vi "FPGA Main High Throughput.vi"() -> ()   [LabVIEW 2015]
doc: "The myRIO v1.1 FPGA Shipping Personality. This personality contains support for:\n- 1 Button\n- 4 LED\n- 6 Analog Input channels with 1 Sample\n- 1 Analog Input channel with N Samples\n- 4 Analog Output channels with 1 Sample\n- 1 Analog Output channel with N Samples\n- 24 Digital I/O channels with 1 Sample\n- 1 Digital Input channel with N Samples\n- 1 Digital Output channel with N Samples"
uses:
  Sub VIs/Utilities/Start Boolean.ctl
  <vilib>/Platform/TimedLoop/XDataNode/timing_clust.ctl
  <vilib>/Platform/TimedLoop/XDataNode/nitl_modes.ctl
  <vilib>/Platform/TimedLoop/XDataNode/wakeup.ctl
  <vilib>/rvi/eio/common/nirviEmuReportErrorAndStop.vi
  <vilib>/rvi/interface/RandomDataEmulation/niFpgaRandomDataHandleErrors.vi
  <vilib>/rvi/Emulation/niFpgaProcessEmulError.vi
  <vilib>/rvi/FIFO/Fifo_Resource/nirvififoEmulationSetSize.vi
  <vilib>/rvi/DataTransferAndStorage/Container/Common/niFpgaContainerGetUniqueNameForEmu.vi
  <vilib>/rvi/FIFO/Fifo_Resource/nirviFifoEmulationQueueMgr.vi
  <instcachedir>/0/nirviFifoEmulationQueueMgr_E5CAEC123FF24DC58D834DCA3CDAA9B5.lvgen/nirviFifoEmulationQueueMgr_E5CAEC123FF24DC58D834DCA3CDAA9B5_003.vi
  <vilib>/rvi/Emulation/niFpgaEmulationIsFPGAContextNoSignature.vi
  <vilib>/rvi/errors/nirviReportUnexpectedCaseInternalError.vi
  <vilib>/rvi/errors/nirviReportUnexpectedCaseInternalError (U32).vi
  <vilib>/rvi/occurrence/nirviWaitOnOccurrenceBase.vi
  <vilib>/rvi/FIFO/Fifo_Resource/nirvififoEmulationReleaseLock.vi
  <vilib>/rvi/FIFO/Fifo_Resource/nirvififoEmulationObtainLock.vi
  <vilib>/rvi/FIFO/Fifo_Resource/nirvififoEmulationCreateLock.vi
  <vilib>/Utility/error.llb/Clear Errors.vi
  <vilib>/rvi/errors/niFpgaSetErrorForExecOnDevCompSimple.vi
  <vilib>/rvi/Emulation/niFpgaSctlEmulationGetInTimedLoop.vi
  <vilib>/rvi/FIFO/Fifo_Resource/nirvififoEmulationDetermineInputValidOut.vi
  <vilib>/rvi/DataTransferAndStorage/Container/Common/niFpgaContainerExecOnDevCompGetState.vi
  <vilib>/rvi/DataTransferAndStorage/Container/Common/niFpgaContainerSetEmuInfo.vi
  <vilib>/rvi/Emulation/niFpgaCriticalErrorInLSC.vi
  <vilib>/rvi/Emulation/niFpgaGetClockAttributes.vi
  <vilib>/rvi/Emulation/niFpgaEmulationReportErrorSimple.vi
  <vilib>/rvi/eio/common/nirviEmuTemplateMethod_errors.vi
  <vilib>/Platform/TimedLoop/XDataNode/XDataNode.xnode
  <vilib>/rvi/DataTransferAndStorage/Container/XNode/niFpgaContainer.xnode
  <vilib>/rvi/FIFO/Fifo_Resource/niFpgaFifoEmulationRefIn.vi
  <vilib>/rvi/LocalResourceManager/LocalResourceManager.xnode
  <vilib>/eio/EIONode/EIONode.xnode
  <vilib>/rvi/interface/RandomDataEmulation/nirviRandomDataFpgaReadWriteTemplate.vi
  <vilib>/rvi/FIFO/Fifo_Resource/nirvififoEmulationWrite.vi
  <vilib>/rvi/FIFO/Fifo_Resource/nirvififoEmulationRead.vi
  <vilib>/Platform/TimedLoop/XDataNode/XDNodeRunTimeDep.lvlib
panel:
  out "AI.B_0.VAL":u16
  out "AI.B_1.VAL":u16
  out "AI.B_2.VAL":u16
  out "AI.B_3.VAL":u16
  in  "AO.B_1.VAL":u16
  in  "AO.B_0.VAL":u16
  out "DIO.B_15:8.IN":u8 format="%08b"
  in  "DIO.B_15:8.DIR":u8 format="%08b"
  in  "DIO.B_15:8.OUT":u8 format="%08b"
  out "DIO.B_7:0.IN":u8 format="%08b"
  in  "DIO.B_7:0.DIR":u8 format="%08b"
  in  "DIO.B_7:0.OUT":u8 format="%08b"
  in  "SYS.SELECTB":u8 format="%08b"
  in  "DO.A_1.IRQ.SELECT":bool
  in  "AO.AudioOut.IRQ.SELECT":bool
  in  "AO.A_0.IRQ.SELECT":bool
  in  "AO.A_0.VAL":u16
  out "AO.A_0.IDL":bool
  out "AO.SYS.STAT":bool
  in  "AO.SYS.GO":T1
  in  "AO.A_1.VAL":u16
  out "AI.AudioIn.IDL":bool
  out "AI.A_0.VAL":u16
  out "AI.AudioIn_R.VAL":u16
  out "AI.AudioIn_L.VAL":u16
  out "AI.A_3.VAL":u16
  out "AI.A_2.VAL":u16
  out "AI.A_1.VAL":u16
  in  "DO.A_1.ClockDivisor":u16 caption="AO LoopRate(Ticks)"
  in  "DI.A_0.ClockDivisor":u16 caption="AO LoopRate(Ticks)"
  out "DO.A_1.IDL":bool
  in  "DI.A_0.ENA":bool
  out "DI.A_0.IDL":bool
  out "DIO.A_15:8.IN":u8 format="%08b"
  in  "DIO.A_15:8.DIR":u8 format="%08b"
  in  "DIO.A_15:8.OUT":u8 format="%08b"
  out "DIO.A_7:0.IN":u8 format="%08b"
  in  "DIO.A_7:0.DIR":u8 format="%08b"
  in  "DIO.A_7:0.OUT":u8 format="%08b"
  in  "AI.AudioIn.SampleRate":u32=40000 caption="Count(Ticks)"
  out "AO.AudioOut.IDL":bool
  in  "AO.AudioOut.SampleRate":u32=40000 caption="AO LoopRate(Ticks)"
  in  "AO.AudioOut_L.VAL":u16
  in  "AO.AudioOut_R.VAL":u16
  out "AI.A_0.IDL":bool
  in  "AI.A_0.SampleRate":u32=40000 caption="Count(Ticks)"
  out "SYS.AI.RDY":bool
  in  "AO.A_0.SampleRate":u32=40000 caption="AO LoopRate(Ticks)"
  out "SYS.RDY":bool
  out "SYS.AUDIN.RDY":bool
  out "SYS.BLOCK.A/AI0.RDY":bool
  in  "SYS.SELECTA":u8 format="%08b"
  out "AI.C_0.VAL":u16
  out "AI.C_1.VAL":u16
  in  "AO.C_0.VAL":u16
  in  "AO.C_1.VAL":u16
  in  "DIO.C_7:0.OUT":u8 format="%08b"
  in  "DIO.C_7:0.DIR":u8 format="%08b"
  out "DIO.C_7:0.IN":u8 format="%08b"
  in  "SYS.SELECTC":u8 format="%08b"
  out "DI.BTN":u8 format="%08b"
  in  "DO.LED3:0":u8 format="%04b"
  out "ACC.X.VAL":u16
  out "ACC.Y.VAL":u16
  out "SYS.ACC.RDY":bool
  out "ACC.Z.VAL":u16
  # "System"
  # "Audio Connector"
  # "Onboard Devices"
  # "Connector A"
  # "Connector B"
  # "Connector C"
  # "Accelerometer"
  # "Audio Input"
  # "Analog Input"
  # "Analog Output"
  # "Digital I/O"
  # "Analog Input"
  # "Analog Output"
  # "Digital I/O"
  # "Analog Input"
  # "Analog Output"
  # "Digital I/O"
  # "Audio Block Input"
  # "Analog Block Output"
  # "Buttons & LEDs"
  # "IO Configuration"
  # "Analog Block Input"
  # "IO Configuration"
  # "Digital Block Input"
  # "Audio Output"
  # "Digital Block Output"
  # "Audio Block Output"
  # "IO Configuration"
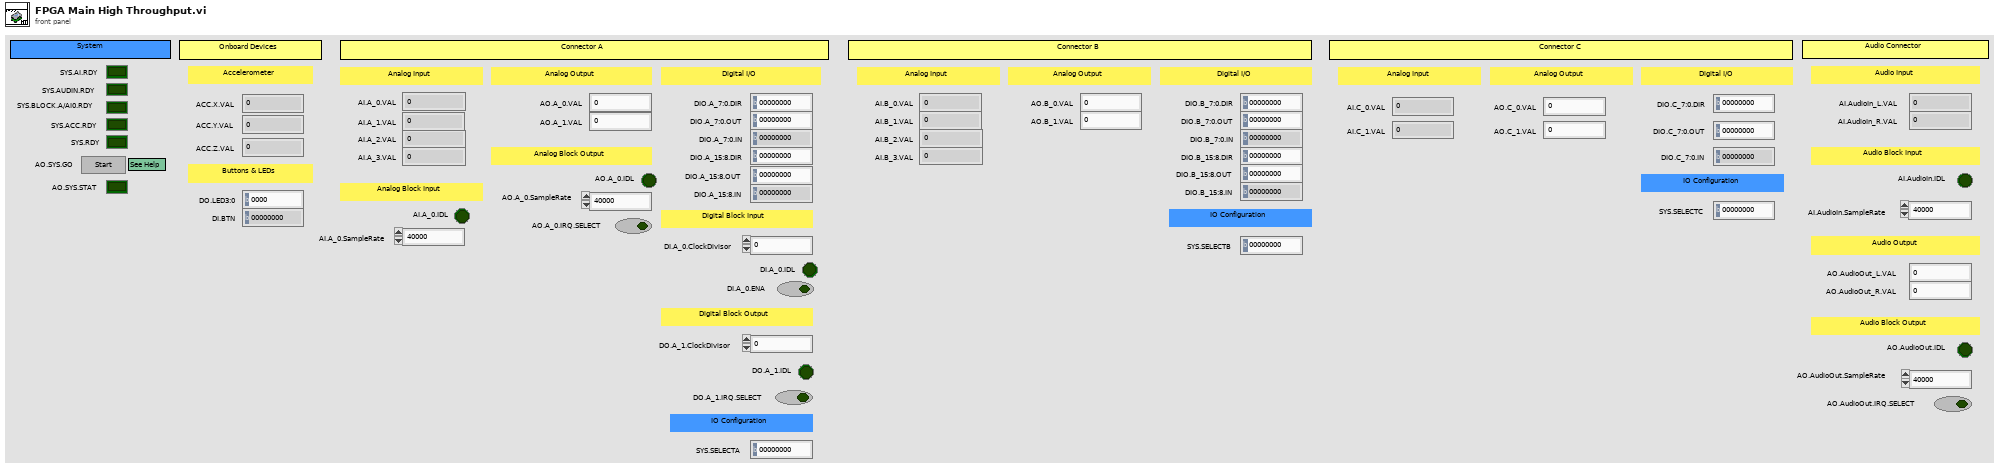
[diagram p1: front panel]
types:
  T1 = typedef "Start Boolean.ctl" = bool
  T2 = typedef "XDNodeRunTimeDep.lvlib/timing_clust.ctl" = cluster{"Expected End [f-1]":u64, "Actual End [f-1]":u64, "Finished Late? [f-1]":bool, "Expected End [i-1]":u64, "Actual End [i-1]":u64, "Finished Late? [i-1]":bool, "Expected Start [i]":u64, "Actual Start [i]":u64, "Expected Start [f]":u64, "Actual Start [f]":u64, "Source Name":string, "Structure Name":string, "Period":i64, "Deadline":i64, "Offset":i64, "Start":i64, "Priority":i32, "Timeout":i32, "Mode":T3, "Wakeup Reason":T4, "Error":errorcluster, "Source Type":string, "Secondary Source Type":string, "Global End Time":u64, "Global Start Time":u64, "Frame Duration":u64, "Iteration Duration":u64, "Assigned CPU":i32, "I/O Scan Engine Mode":u32}
  T3 = typedef "XDNodeRunTimeDep.lvlib/nitl_modes.ctl" = enum32{"No Change", "Process missed periods, maintain original phase", "Discard missed periods, maintain original phase", "Process missed periods, ignore original phase", "Discard missed periods, ignore original phase"}
  T4 = typedef "XDNodeRunTimeDep.lvlib/wakeup.ctl" = enum32{"Normal", "Aborted", "Asynchronous wakeup", "Timing source error", "Timed loop error", "Timeout"}
diagram:
  # "The accelerometer nodes take some time before the FPGA can first read the values. This is because it takes time to read from the accelerometer. An iteration of the While Loop will not complete until the accelerometer values have been read.\n\nAfter the completion of the first iteration of the While Loop, all indicators have valid values."
  # "This loop fetches one element from AudioOut DMA FIFO at one time, splits the data into AudioOut/Left and AudioOut/Right data and writes the data to the audio left and right channels. \nThis loop pushes IRQ to Write Finished Queue every time when finishes writing."
  # "This loop fetches on element from A.AO0 DMA FIFO at one time and writes to channel A/AO0. This loop pushes IRQ to Write Finished Queue every time when it finishes writing."
  # "The analog output nodes take some time before the FPGA write the values to the pins. The GO and STAT registers are used to handshake between the FPGA and host. When the host wants the values to be written, the host sets the GO register to TRUE. If the host reads the STAT register before setting the value of the GO register, it can wait for the value of the STAT register to invert. The value inversion tells the host that the output values have been written."
  # "This loop acquires data from AudioIn channels and combines AudioIn/Left and AudioIn/Right data into one data and writes one element of data to AudioIn DMA FIFO at one time."
  # "This loop acquires data from channel A/AI0 and writes one element of data to A.AI0 DMA FIFO at one time."
  # "Note: On some hardware a \"ghosting effect\" may occur on any unconnected AI channels. For example, if channel AI0 is connected and channels AI1~AI7 are not connected the the value read at AI0 may be seen on indicators AI1~AI7. This is common for hardware that use a multiplexed (MUXed) Analog-to-Digital converter (ADC), because the input analog signal is used to charge a capacitor which does not discharge before the unconnected channel is read.\n\nYou can hide the \"ghosting effect\" by using an mask register. This register is used to decide when the indicator should be updated."
  # "The analog input nodes take some time before the FPGA can first read the values. This is because it takes time to set up the Analog-to-Digital converter (ADC) and convert the first reading. An iteration of the While Loop will not complete until all the analog input channels have been sampled.\n\nAfter the completion of the first iteration of the While Loop, all indicators have valid values."
  # "Because Write Finished Queue cannot be shared between a single-cycle Timed Loop and any other loop, DIO Write Finished Queue is required. Use this queue to transfer IRQ from DIO to IRQ Write Finished Queue."
  # "This loop retrieves the IRQ number from Write Finished Queue and send IRQ to the RT side. \n\nWhen the FPGA finishes writing n samples, it pushes an IRQ number to Write Finished Queue. The RT side waits for the IRQ after it writes n samples to the Direct Memory Access (DMA) channel. Only when the RT side recieves the IRQ, it sends another n samples.\n\nAO               IRQ: 9, 12\nAudioOut   IRQ: 10, 13\nDO               IRQ: 11, 14"
  # "NOTE: The SYS.RDY Boolean MUST exist and must become TRUE at some point. Otherwise, the myRIO VIs will not function correctly."
  # "There is some delay between the time when the FPGA code starts and the time when the analog inputs, accelerometer, and scaling values outputs are valid. If the host wants to ensure that there are valid values in theses registers it should wait for each subsystem to finish its initialization process. \n\nWhen all subsystems have finished initializinig, the SYS.RDY indicator turns true. The host can poll the SYS.RDY indicator to determine the status of the FPGA. Alternatively, the host can poll the individual SYS.xx.RDY indicators to determine the status of the individual subsystems.\n\nThis loop continues indefinitely, essentially making SYS.RDY a read-only register."
  n1 = while {
    stop <- FALSE stop-if-true
    # "Host Synchronization"
    n2 = local read "SYS.BLOCK.A/AI0.RDY"() -> (w11:bool)
    n3 = local read "SYS.AUDIN.RDY"() -> (w12:bool)
    n4 = local read "SYS.ACC.RDY"() -> (w9:bool)
    n5 = local read "SYS.AI.RDY"() -> (w14:bool)
    n6 = Compound Arithmetic op=AND(w14, w12, w11, w9) -> (→"SYS.RDY":bool)
  }
  n7 = while {
    stop <- FALSE stop-if-true
    # "Send Write Finished IRQ"
    n8 = xnode ("FIFO Read")("Timeout"=-1) -> ("Element"=w17:u8)  [unwired: 1 in, 2 out]
    n9 = call <vilib>:"niFPGA Interrupt.vi"("IRQ Number (0)"=w17) -> ()  [unwired: 2 in]
  }
  n10 = xnode "VI-Defined FIFO Configuration"() -> ()  [unwired: 1 out]
  n11 = while {
    stop <- FALSE stop-if-true
    # "DIO Write Finished IRQ"
    n12 = feedback #1(u8 0 ("Element")) -> (w20:u8)
    n13 = feedback #2(FALSE ("Timed Out?")) -> (w24:bool)
    n14 = case shown="False" w24 {
      tunnel: [w26 w28] -> w21
      tunnel: w20 -> [_ w28]
      frame False {
        n15 = xnode ("FIFO Method Node")("Timeout"=-1) -> ("Element"=w26:u8)  [unwired: 1 in, 2 out]
      }
      frame True {
      }
    }
    n16 = feedback-in #1(w21) -> ()
    n17 = xnode ("FIFO Method Node")("Element"=w21, "Timeout"=0) -> ("Timed Out?"=w22:bool)  [unwired: 1 in, 1 out]
    n18 = feedback-in #2(w22) -> ()
  }
  n19 = while {
    i -> [w37]
    stop <- FALSE stop-if-true
    # "Sets the sample rate of the analog \ninput signal acquisition to 12 kHz."
    # "Analog Input"
    n20 = xnode "FPGA I/O Node"() -> ("ConnectorA/AI1"=→"AI.A_1.VAL":u16, "ConnectorA/AI2"=→"AI.A_2.VAL":u16, "ConnectorA/AI3"=→"AI.A_3.VAL":u16, "ConnectorB/AI0"=→"AI.B_0.VAL":u16, "ConnectorB/AI1"=→"AI.B_1.VAL":u16, "ConnectorB/AI2"=→"AI.B_2.VAL":u16, "ConnectorB/AI3"=→"AI.B_3.VAL":u16, "ConnectorC/AI0"=w34:i16, "ConnectorC/AI1"=w33:i16)  [unwired: 9 in, 9 out]
    n21 = Greater Than 0?(x=w37) -> (x > 0?=→"SYS.AI.RDY":bool)
    n22 = To Unsigned Word Integer(number=w34) -> (unsigned 16bit integer=→"AI.C_0.VAL":u16)
    n23 = To Unsigned Word Integer(number=w33) -> (unsigned 16bit integer=→"AI.C_1.VAL":u16)
    n24 = call "Loop Timer2"("Count(Ticks)"=u32 3333) -> ()  [unwired: 1 out]
  }
  n25 = while {
    i -> [w45]
    stop <- FALSE stop-if-true
    # "A/AI0 Input N Samples Read"
    n26 = xnode "FPGA I/O Node"() -> ("ConnectorA/AI0"=w46:u16)  [unwired: 1 in, 1 out]
    "AI.A_0.VAL" <- w46
    n27 = Greater Than 0?(x=w45) -> (x > 0?=→"SYS.BLOCK.A/AI0.RDY":bool)
    n28 = xnode ("FIFO Method Node")("Element"=w46, "Timeout"=0) -> ("Timed Out?"=→"AI.A_0.IDL":bool)  [unwired: 1 in, 1 out]
    n29 = call "Loop Timer5"("Count(Ticks)"="AI.A_0.SampleRate") -> ()  [unwired: 1 out]
  }
  n30 = while {
    i -> [w52]
    stop <- FALSE stop-if-true
    # "Audio Input N Samples Read"
    n31 = xnode "FPGA I/O Node"() -> ("AudioIn/Left"=w59:i16, "AudioIn/Right"=w58:i16)  [unwired: 2 in, 2 out]
    n32 = Greater Than 0?(x=w52) -> (x > 0?=→"SYS.AUDIN.RDY":bool)
    n33 = To Unsigned Word Integer(number=w59) -> (unsigned 16bit integer=w57:u16)
    "AI.AudioIn_L.VAL" <- w57
    n34 = To Unsigned Word Integer(number=w58) -> (unsigned 16bit integer=w56:u16)
    "AI.AudioIn_R.VAL" <- w56
    n35 = Join Numbers(hi=w57, lo=w56) -> ((hi.lo)=w61:u32)
    n36 = xnode ("FIFO Method Node")("Element"=w61, "Timeout"=0) -> ("Timed Out?"=→"AI.AudioIn.IDL":bool)  [unwired: 1 in, 1 out]
    n37 = call "Loop Timer3"("Count(Ticks)"="AI.AudioIn.SampleRate") -> ()  [unwired: 1 out]
  }
  n38 = while {
    stop <- FALSE stop-if-true
    # "Set the sample rate of the analog input \nsignal acquisition to 12 kHz."
    # "Analog Output"
    n39 = feedback #3(FALSE) -> (w72:bool)
    n40 = case shown="True" "AO.SYS.GO" {
      tunnel: "AO.A_0.VAL" -> [_ w91]
      tunnel: "AO.A_1.VAL" -> [_ w90]
      tunnel: w72 -> [w76 w89]
      tunnel: [w76 w87] -> w71
      tunnel: "AO.AudioOut_L.VAL" -> [_ w84]
      tunnel: "AO.AudioOut_R.VAL" -> [_ w83]
      tunnel: "AO.C_0.VAL" -> [_ w81]
      tunnel: "AO.C_1.VAL" -> [_ w80]
      tunnel: "AO.B_0.VAL" -> [_ w78]
      tunnel: "AO.B_1.VAL" -> [_ w77]
      frame False {
      }
      frame True {
        n41 = To Word Integer(number=w81) -> (16bit integer=w82:i16)
        n42 = To Word Integer(number=w80) -> (16bit integer=w79:i16)
        n43 = To Word Integer(number=w84) -> (16bit integer=w86:i16)
        n44 = To Word Integer(number=w83) -> (16bit integer=w85:i16)
        n45 = flat-sequence {
          tunnel: w91 -> [w100]
          tunnel: w90 -> [w99]
          tunnel: w82 -> [w98]
          tunnel: w89 -> [w97]
          tunnel: [w97] -> w88
          tunnel: w86 -> [w96]
          tunnel: w85 -> [w95]
          tunnel: w79 -> [w94]
          tunnel: w78 -> [w93]
          tunnel: w77 -> [w92]
          tunnel: w88 -> [w102]
          tunnel: [w101] -> w87
          frame #0 {
            n46 = xnode "FPGA I/O Node"("ConnectorA/AO0"=w100, "ConnectorA/AO1"=w99, "ConnectorB/AO0"=w93, "ConnectorB/AO1"=w92, "ConnectorC/AO0"=w98, "ConnectorC/AO1"=w94, "AudioOut/Left"=w96, "AudioOut/Right"=w95) -> ()  [unwired: 8 in, 8 out]
          }
          frame #1 {
            n47 = Not(x=w102) -> (.not. x?=w101:bool)
          }
        }
      }
    }
    "AO.SYS.STAT" <- w71
    n48 = feedback-in #3(w71) -> ()
    n49 = call "Loop Timer"("Count(Ticks)"=u32 3333) -> ()  [unwired: 1 out]
  }
  n50 = while {
    stop <- FALSE stop-if-true
    w104 = u8 12  # IRQ Num_Non Wait
    w106 = u8 9  # IRQ Num_Wait
    # "A/AO0 Output N Samples Write"
    n51 = xnode ("FIFO Method Node")("Timeout"=0) -> ("Element"=w114:u16, "Timed Out?"=w112:bool)  [unwired: 1 in, 1 out]
    "AO.A_0.IDL" <- w112
    n52 = call "Rising Edge Trigger.vi"("Signal"=w112) -> ("Trigger?"=w108:bool)
    n53 = Select(t=w106, s="AO.A_0.IRQ.SELECT", f=w104) -> (s? t:f=w103:u8)
    n54 = case shown="False" w112 {
      tunnel: w114 -> [w121 _]
      frame False {
        n55 = xnode "FPGA I/O Node"("ConnectorA/AO0"=w121) -> ()  [unwired: 1 in, 1 out]
      }
      frame True {
      }
    }
    n56 = case shown="False" w112 {
      tunnel: w114 -> [w122 _]
      frame False {
        # "Save the last value."
        n57 = local write "AO.A_0.VAL"(w122) -> ()
      }
      frame True {
      }
    }
    n58 = feedback #4(FALSE ("Timed Out?")) -> (w110:bool)
    n59 = Or(x=w108, y=w110) -> (x .or. y?=w107:bool)
    n60 = case shown="True" w107 {
      selector: w107 -> [w117 _]
      tunnel: [w117 w120] -> w111
      tunnel: w103 -> [_ w118]
      frame False {
      }
      frame True {
        n61 = xnode ("FIFO Write")("Element"=w118, "Timeout"=0) -> ("Timed Out?"=w120:bool)  [unwired: 1 in, 1 out]
      }
    }
    n62 = feedback-in #4(w111) -> ()
    n63 = call "Loop Timer6"("Count(Ticks)"="AO.A_0.SampleRate") -> ()  [unwired: 1 out]
  }
  n64 = while {
    stop <- FALSE stop-if-true
    w125 = u8 10  # IRQ Num_Wait
    w126 = u8 13  # IRQ Num_Non Wait
    # "Audio Output N Samples Write"
    n65 = xnode ("FIFO Method Node")("Timeout"=0) -> ("Element"=w136:u32, "Timed Out?"=w132:bool)  [unwired: 1 in, 1 out]
    "AO.AudioOut.IDL" <- w132
    n66 = Split Number(x=w136) -> (hi(x)=w135:u16, lo(x)=w134:u16)
    n67 = call "Rising Edge Trigger.vi"("Signal"=w132) -> ("Trigger?"=w129:bool)
    n68 = Select(t=w125, s="AO.AudioOut.IRQ.SELECT", f=w126) -> (s? t:f=w123:u8)
    n69 = case shown="False" w132 {
      tunnel: w135 -> [w148 _]
      tunnel: w134 -> [w147 _]
      frame False {
        n70 = To Word Integer(number=w148) -> (16bit integer=w146:i16)
        n71 = To Word Integer(number=w147) -> (16bit integer=w145:i16)
        n72 = xnode "FPGA I/O Node"("AudioOut/Left"=w146, "AudioOut/Right"=w145) -> ()  [unwired: 2 in, 2 out]
      }
      frame True {
      }
    }
    n73 = case shown="False" w132 {
      tunnel: w134 -> [w144 _]
      tunnel: w135 -> [w143 _]
      frame False {
        # "Save the last value."
        n74 = local write "AO.AudioOut_R.VAL"(w144) -> ()
        n75 = local write "AO.AudioOut_L.VAL"(w143) -> ()
      }
      frame True {
      }
    }
    n76 = feedback #5(FALSE ("Timed Out?")) -> (w128:bool)
    n77 = Or(x=w129, y=w128) -> (x .or. y?=w127:bool)
    n78 = case shown="True" w127 {
      selector: w127 -> [w139 _]
      tunnel: [w139 w141] -> w130
      tunnel: w123 -> [_ w140]
      frame False {
      }
      frame True {
        n79 = xnode ("FIFO Write")("Element"=w140, "Timeout"=0) -> ("Timed Out?"=w141:bool)  [unwired: 1 in, 1 out]
      }
    }
    n80 = feedback-in #5(w130) -> ()
    n81 = call "Loop Timer4"("Count(Ticks)"="AO.AudioOut.SampleRate") -> ()  [unwired: 1 out]
  }
  n82 = while {
    i -> [w153]
    stop <- FALSE stop-if-true
    # "Onboard Accelerometer"
    n83 = xnode "FPGA I/O Node"() -> ("AccelerationX"=w156:i16, "AccelerationY"=w155:i16, "AccelerationZ"=w154:i16)  [unwired: 3 in, 3 out]
    n84 = Greater Than 0?(x=w153) -> (x > 0?=→"SYS.ACC.RDY":bool)
    n85 = To Unsigned Word Integer(number=w156) -> (unsigned 16bit integer=→"ACC.X.VAL":u16)
    n86 = To Unsigned Word Integer(number=w155) -> (unsigned 16bit integer=→"ACC.Y.VAL":u16)
    n87 = To Unsigned Word Integer(number=w154) -> (unsigned 16bit integer=→"ACC.Z.VAL":u16)
  }
  n88 = node-c288() -> (w2:T2)  [unwired: 1 in]
  n89 = timed-loop {
    timing: w2 -> [_]
    timing-out: [_] -> w1
    stop <- _ stop-if-true
    # "Onboard DIO"
    n90 = xnode "FPGA I/O Node"() -> ("Button0"=w166:bool)  [unwired: 1 in, 1 out]
    n91 = Number To Boolean Array(number="DO.LED3:0") -> (Boolean array=w162:bool[])
    n92 = Build Array(w166) -> (w165:bool[])
    n93 = Index Array(array=w162) -> (element #1=w161:bool, element #2=w160:bool, element #3=w159:bool, element #4=w158:bool)  [unwired: 4 in]
    n94 = Boolean Array To Number(Boolean array=w165) -> (number=→"DI.BTN":u8)
    n95 = xnode "FPGA I/O Node"("LED0"=w161, "LED1"=w160, "LED2"=w159, "LED3"=w158) -> ()  [unwired: 4 in, 4 out]
  }
  n96 = node-c288(w1) -> ()
  n97 = node-c288() -> (w8:T2)  [unwired: 1 in]
  n98 = timed-loop {
    timing: w8 -> [_]
    timing-out: [_] -> w7
    stop <- _ stop-if-true
    w178 = u8 14  # IRQ Num_Non Wait
    w177 = u8 11  # IRQ Num_Wait
    # "DO Block Write"
    # "DI Block Read"
    # "Connector A  DIO"
    n99 = xnode "VI-Defined FIFO Configuration"() -> ("FIFO Out"=w169:refnum<k21>)
    n100 = Number To Boolean Array(number="DIO.A_7:0.DIR") -> (Boolean array=w214:bool[])
    n101 = Number To Boolean Array(number="DIO.A_7:0.OUT") -> (Boolean array=w220:bool[])
    n102 = Index Array(array=w214) -> (element #1=w197:bool, element #2=w182:bool, element #3=w194:bool, element #4=w192:bool, element #5=w213:bool, element #6=w212:bool, element #7=w211:bool, element #8=w210:bool)  [unwired: 8 in]
    n103 = Index Array(array=w220) -> (element #1=w199:bool, element #2=w183:bool, element #3=w195:bool, element #4=w193:bool, element #5=w218:bool, element #6=w217:bool, element #7=w216:bool, element #8=w215:bool)  [unwired: 8 in]
    n104 = call "DIO 1-bit.vi"("DIR"=w192, "OUT"=w193, "DIO Refnum"=refnum<k21> "ConnectorA/DIO3" ("DIO/PWM")) -> ("IN"=w190:bool)  [unwired: 8 in]
    n105 = call "DIO 1-bit.vi"("DIR"=w194, "OUT"=w195, "DIO Refnum"=refnum<k21> "ConnectorA/DIO2") -> ("IN"=w191:bool)  [unwired: 8 in]
    n106 = call "DIO Block Read.vi"("ENA"="DI.A_0.ENA", "Divisor"="DI.A_0.ClockDivisor", "DIR"=w197, "OUT"=w199, "FIFO In"=refnum<k21> "A.DI0 DMA", "DIO Refnum"=refnum<k21> "ConnectorA/DIO0" ("DIO.0/QE.A")) -> ("Timed Out?"=→"DI.A_0.IDL":bool, "IN"=w198:bool)  [unwired: 4 in]
    n107 = call "DIO Block Write.vi"("Divisor"="DO.A_1.ClockDivisor", "DIR"=w182, "OUT"=w183, "DMA FIFO In"=refnum<k21> "A.DO1 DMA", "DIO Refnum"=refnum<k21> "ConnectorA/DIO1" ("DIO.1/QE.B")) -> ("Timed Out?"=w170:bool, "IN"=w196:bool)  [unwired: 5 in]
    "DO.A_1.IDL" <- w170
    n108 = call "Rising Edge Trigger.vi"("Signal"=w170) -> ("Trigger?"=w174:bool)
    n109 = Select(t=w177, s="DO.A_1.IRQ.SELECT", f=w178) -> (s? t:f=w179:u8)
    n110 = feedback #6(FALSE ("Timed Out?")) -> (w173:bool)
    n111 = Or(x=w174, y=w173) -> (x .or. y?=w172:bool)
    n112 = case shown="True" w172 {
      selector: w172 -> [w235 _]
      tunnel: [w235 w237] -> w175
      tunnel: w169 -> [_ w238]
      tunnel: w179 -> [_ w236]
      frame False {
      }
      frame True {
        n113 = xnode ("FIFO Write")("Element"=w236, "Timeout"=0, "FIFO In"=w238) -> ("Timed Out?"=w237:bool)  [unwired: 1 out]
      }
    }
    n114 = feedback-in #6(w175) -> ()
    n115 = call "DIO 1-bit.vi"("DIR"=w213, "OUT"=w218, "DIO Refnum"=refnum<k21> "ConnectorA/DIO4" ("DIO.0/QE.A")) -> ("IN"=w209:bool)  [unwired: 8 in]
    n116 = call "DIO 1-bit.vi"("DIR"=w211, "OUT"=w216, "DIO Refnum"=refnum<k21> "ConnectorA/DIO6") -> ("IN"=w207:bool)  [unwired: 8 in]
    n117 = call "DIO 1-bit.vi"("DIR"=w210, "OUT"=w215, "DIO Refnum"=refnum<k21> "ConnectorA/DIO7" ("DIO/PWM")) -> ("IN"=w206:bool)  [unwired: 8 in]
    n118 = call "DIO 1-bit.vi"("DIR"=w212, "OUT"=w217, "DIO Refnum"=refnum<k21> "ConnectorA/DIO5" ("DIO.1/QE.B")) -> ("IN"=w208:bool)  [unwired: 8 in]
    n119 = Build Array(w198, w196, w191, w190, w209, w208, w207, w206) -> (w205:bool[])
    n120 = Boolean Array To Number(Boolean array=w205) -> (number=→"DIO.A_7:0.IN":u8)
    n121 = call "DIO 8-bit.vi"("DIO 7 Refnum"=refnum<k21> "ConnectorA/DIO15" ("DIO.1/I2C.SCL"), "DIO 0 Refnum"=refnum<k21> "ConnectorA/DIO8" ("DIO/PWM"), "DIO 6 Refnum"=refnum<k21> "ConnectorA/DIO14" ("DIO.0/I2C.SDA"), "DIO 1 Refnum"=refnum<k21> "ConnectorA/DIO9" ("DIO/PWM"), "DIO 5 Refnum"=refnum<k21> "ConnectorA/DIO13" ("DIO Refnum"), "DIO 2 Refnum"=refnum<k21> "ConnectorA/DIO10" ("DIO/PWM"), "DIO 4 Refnum"=refnum<k21> "ConnectorA/DIO12" ("DIO.1/QE.B"), "DIR 7:0"="DIO.A_15:8.DIR", "OUT 7:0"="DIO.A_15:8.OUT", "DIO 3 Refnum"=refnum<k21> "ConnectorA/DIO11" ("DIO.0/QE.A")) -> ("IN 7:0"=→"DIO.A_15:8.IN":u8)  [unwired: 1 in]
  }
  n122 = node-c288(w7) -> ()
  n123 = node-c288() -> (w4:T2)  [unwired: 1 in]
  n124 = timed-loop {
    timing: w4 -> [_]
    timing-out: [_] -> w3
    stop <- _ stop-if-true
    # "Connector B  DIO"
    n125 = call "DIO 8-bit.vi"("DIO 7 Refnum"=refnum<k21> "ConnectorB/DIO7" ("DIO.2/SPI.SCLK"), "DIO 0 Refnum"=refnum<k21> "ConnectorB/DIO0" ("DIO0 Refnum"), "DIO 6 Refnum"=refnum<k21> "ConnectorB/DIO6" ("DIO.1/SPI.MOSI"), "DIO 1 Refnum"=refnum<k21> "ConnectorB/DIO1" ("DIO1 Refnum"), "DIO 5 Refnum"=refnum<k21> "ConnectorB/DIO5" ("DIO.0/SPI.MISO"), "DIO 2 Refnum"=refnum<k21> "ConnectorB/DIO2" ("DIO2 Refnum"), "DIO 4 Refnum"=refnum<k21> "ConnectorB/DIO4" ("DIO Refnum"), "DIR 7:0"="DIO.B_7:0.DIR", "OUT 7:0"="DIO.B_7:0.OUT", "DIO 3 Refnum"=refnum<k21> "ConnectorB/DIO3" ("DIO3 Refnum")) -> ("IN 7:0"=→"DIO.B_7:0.IN":u8)  [unwired: 1 in]
    n126 = call "DIO 8-bit.vi"("DIO 7 Refnum"=refnum<k21> "ConnectorB/DIO15" ("DIO.2/SPI.SCLK"), "DIO 0 Refnum"=refnum<k21> "ConnectorB/DIO8" ("DIO0 Refnum"), "DIO 6 Refnum"=refnum<k21> "ConnectorB/DIO14" ("DIO.1/SPI.MOSI"), "DIO 1 Refnum"=refnum<k21> "ConnectorB/DIO9" ("DIO1 Refnum"), "DIO 5 Refnum"=refnum<k21> "ConnectorB/DIO13" ("DIO.0/SPI.MISO"), "DIO 2 Refnum"=refnum<k21> "ConnectorB/DIO10" ("DIO2 Refnum"), "DIO 4 Refnum"=refnum<k21> "ConnectorB/DIO12" ("DIO Refnum"), "DIR 7:0"="DIO.B_15:8.DIR", "OUT 7:0"="DIO.B_15:8.OUT", "DIO 3 Refnum"=refnum<k21> "ConnectorB/DIO11" ("DIO3 Refnum")) -> ("IN 7:0"=→"DIO.B_15:8.IN":u8)  [unwired: 1 in]
  }
  n127 = node-c288(w3) -> ()
  n128 = node-c288() -> (w6:T2)  [unwired: 1 in]
  n129 = timed-loop {
    timing: w6 -> [_]
    timing-out: [_] -> w5
    stop <- _ stop-if-true
    # "Connector C  DIO"
    n130 = call "DIO 8-bit.vi"("DIO 7 Refnum"=refnum<k21> "ConnectorC/DIO7" ("DIO.2/SPI.SCLK"), "DIO 0 Refnum"=refnum<k21> "ConnectorC/DIO0" ("DIO0 Refnum"), "DIO 6 Refnum"=refnum<k21> "ConnectorC/DIO6" ("DIO.1/SPI.MOSI"), "DIO 1 Refnum"=refnum<k21> "ConnectorC/DIO1" ("DIO1 Refnum"), "DIO 5 Refnum"=refnum<k21> "ConnectorC/DIO5" ("DIO.0/SPI.MISO"), "DIO 2 Refnum"=refnum<k21> "ConnectorC/DIO2" ("DIO2 Refnum"), "DIO 4 Refnum"=refnum<k21> "ConnectorC/DIO4" ("DIO Refnum"), "DIR 7:0"="DIO.C_7:0.DIR", "OUT 7:0"="DIO.C_7:0.OUT", "DIO 3 Refnum"=refnum<k21> "ConnectorC/DIO3" ("DIO3 Refnum")) -> ("IN 7:0"=→"DIO.C_7:0.IN":u8)  [unwired: 1 in]
  }
  n131 = node-c288(w5) -> ()
